vi "GUI_HTU_Chicane.vi"() -> ()   [LabVIEW 2013]
uses:
  Shared/GUI_Template/GUI_master/tcp_new_data_event.ctl
  Shared/GUI_Template/GUI_master/tcp new data cluster.ctl
panel:
  in  "DigitalOutput.Channel 5::4":enum16{"on", "off"}(ring) caption="ChicaneSlits\nplunger"
  in  "GUIdevice 4":string="U_Valve_Daq"
  in  "Ch1Ax2MovePos::3":bool=TRUE caption="Blank Button"
  in  "Ch1Ax2MoveNeg::3":bool=TRUE caption="Blank Button"
  in  "Ch1Ax1MovePos::3":bool=TRUE caption="Blank Button"
  in  "Ch1Ax1MoveNeg::3":bool=TRUE caption="Blank Button"
  in  "Ch1Ax2StepSize::3":dbl caption="High E Step size (mm)" min=0.01 max=2.0
  in  "Ch1Ax1StepSize::3":dbl caption="Low E Step size (mm)" min=0.01 max=2.0
  in  "Voltage::2":dbl caption="Inner \nVoltage" min=0.0 max=15.0
  in  "Current::2":dbl caption="Inner \nCurrent" min=-12.0 max=12.0
  in  "Voltage::1":dbl caption="Outer \nVoltage" min=0.0 max=15.0
  in  "Current::1":dbl caption="Outer \nCurrent" min=-12.0 max=12.0
  in  "Enable_Output::2":bool=TRUE caption="Blank Button"
  in  "Enable_Output::1":bool=TRUE caption="Blank Button"
  in  "GUIdevice 3":string="U_ChicaneMotors"
  in  "Enable_Output::2":enum16{"on", "off"}(ring) caption="Enable inner"
  in  "Enable_Output::1":enum16{"on", "off"}(ring) caption="Enable outer"
  in  "RunList::2":enum16{"on", "off"}(ring) caption="Run List \nInner Pair"
  in  "RunList::1":enum16{"on", "off"}(ring) caption="Run List \nOuter Pair"
  in  "LoadList::2":enum16{"on", "off"}(ring) caption="Load List \nInner Pair"
  in  "LoadList::1":enum16{"on", "off"}(ring) caption="Load List \nOuter Pair"
  out "Chart":cluster{"Value":dbl, "Value":dbl}(graph)
  in  "ApplyChicaneSettings":bool
  in  "Energy (MeV)":dbl=100.0
  in  "R56 (um)":dbl
  out "Offset (mm)":dbl
  out "Width of 2%  (mm)":dbl
  out "SetCurrent":dbl
  in  "CalculateChicaneSettings":bool
  out "error IO 2":errorcluster
  out "tcp data event":T1
  in  "UDP error message":string
  in  "GUIdevice 2":string="U_ChicaneInner"
  in  "GUIdevice 1":string="U_ChicaneOuter"
  in  "stop":bool
  # "HTU Chicane"
  # "Chicane slit operation"
  # "Energy"
  # "Outer pair"
  # "Inner pair"
  # "Enable"
  # "Current"
  # "Move High E direction"
  # "Voltage"
  # "Move Low E direction"
  # "Degaussing"
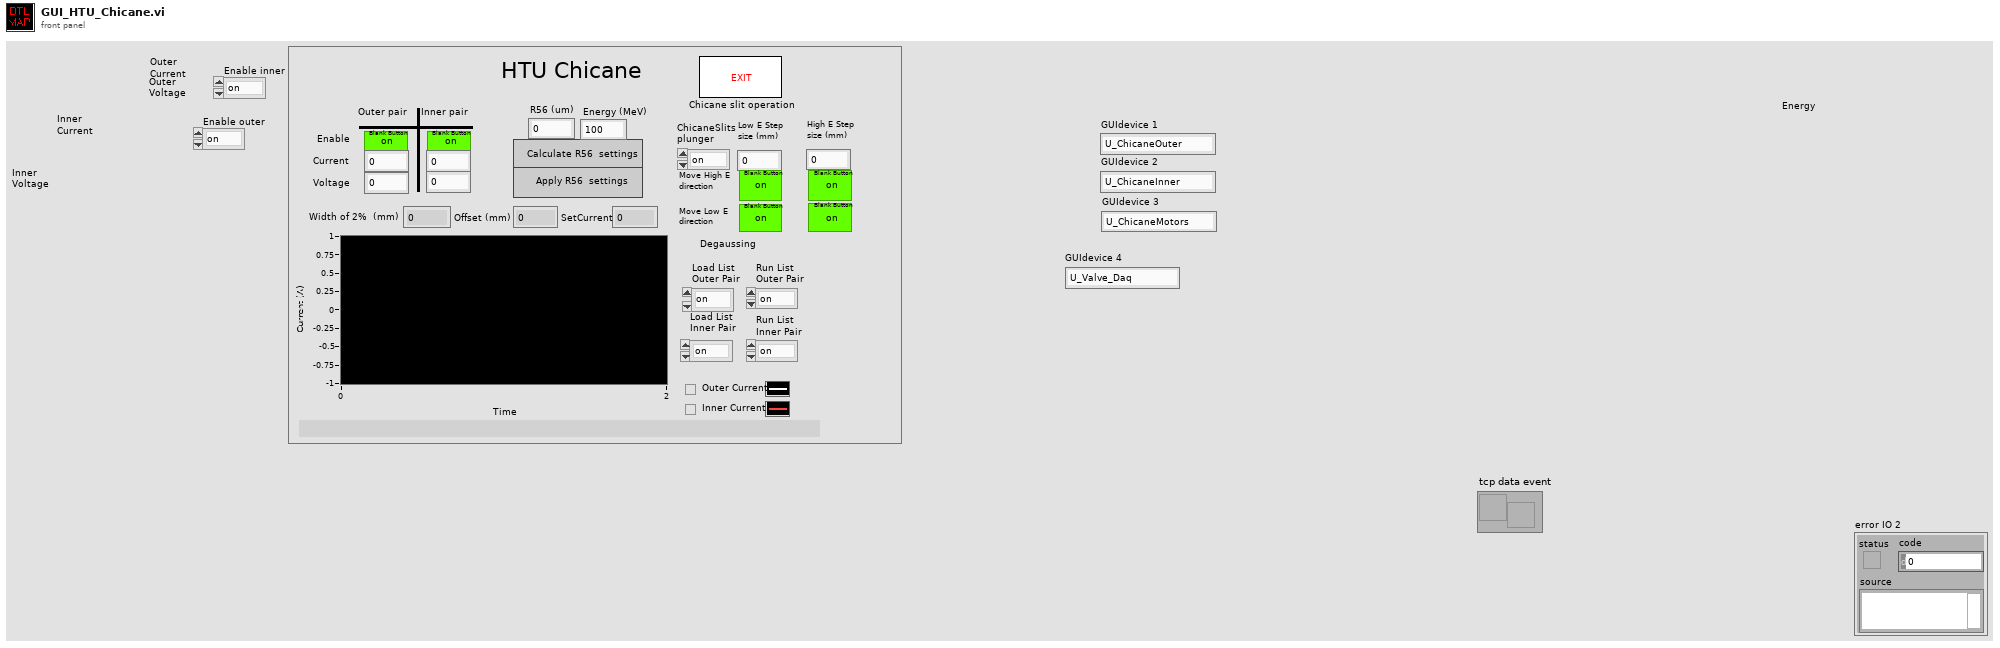
[diagram p1: front panel]
types:
  T1 = typedef "tcp_new_data_event.ctl" = refnum<user-event>
  T2 = typedef "tcp new data cluster.ctl" = cluster{"EventEnum":enum16{"new data", "connection status update"}, "Device name":string}
  T3 = enum32{"invalid app kind", "Development System", "Run Time System", "Student Edition", "Embedded LabVIEW", "Evaluation", "Custom"}
  T4 = enum32{"Invalid", "Standard", "Closed", "Hidden", "Minimized", "Maximized"}
  T5 = cluster{"Core":cluster{"Current VI Reference":refnum<vi>, "Close Panel on Exit?":bool}, "CalculateChicanceSettings":bool, "ApplyChicanceSettings":bool, "CurrentGraph1":dbl[][], "last chart update tck":i32}
  T6 = cluster{"Current VI Reference":refnum<vi>, "Close Panel on Exit?":bool}
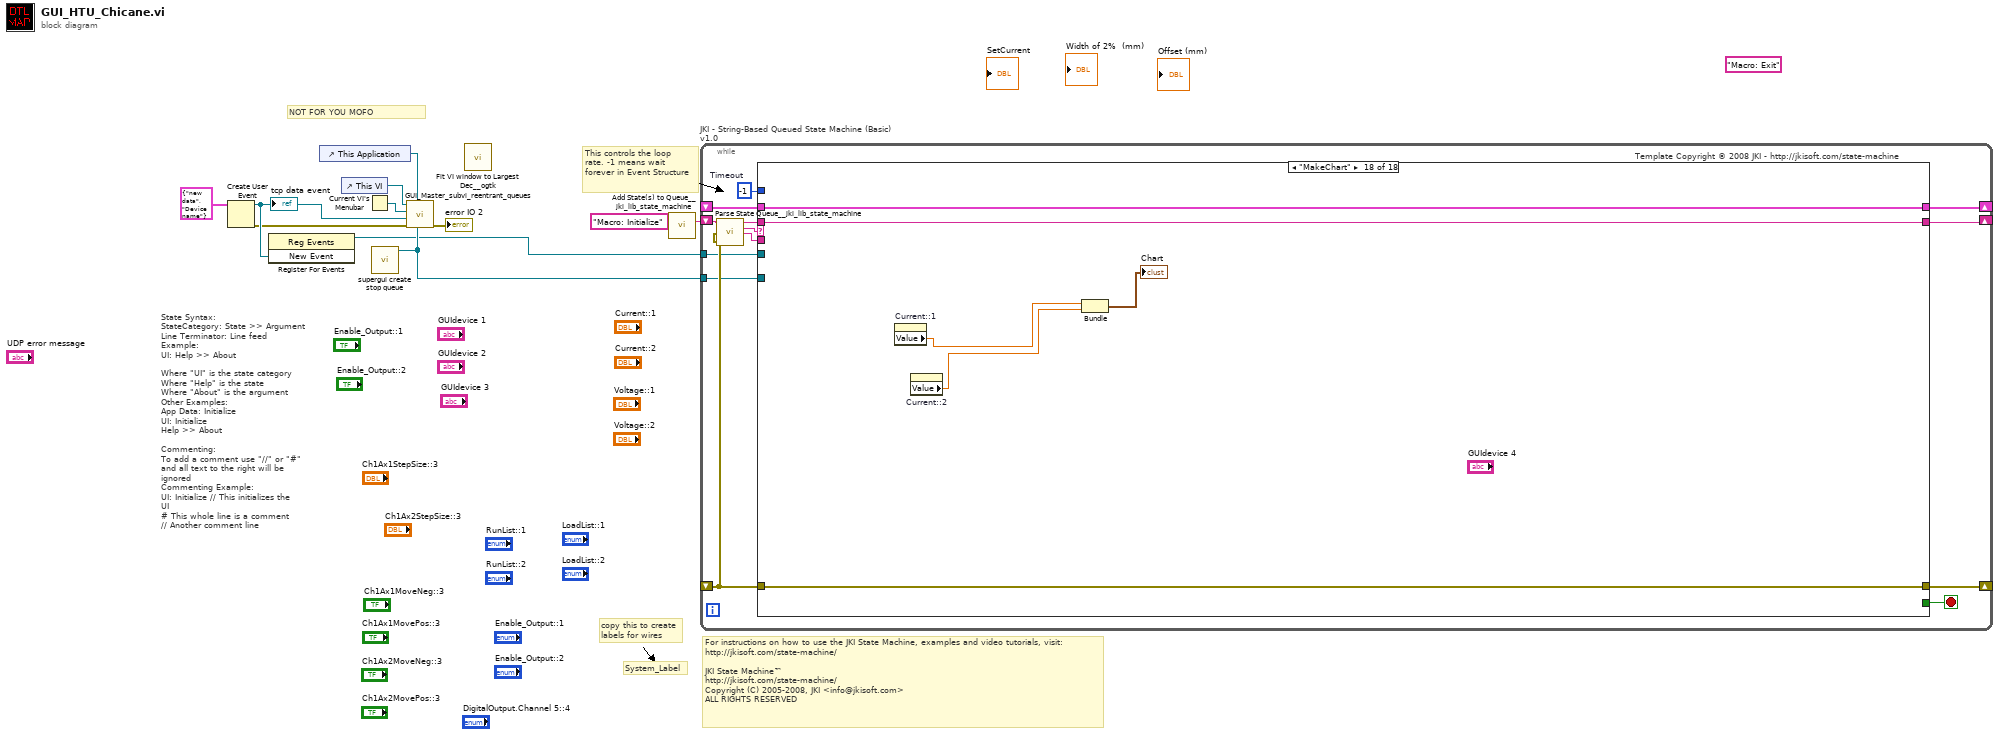
[diagram p0: block diagram]
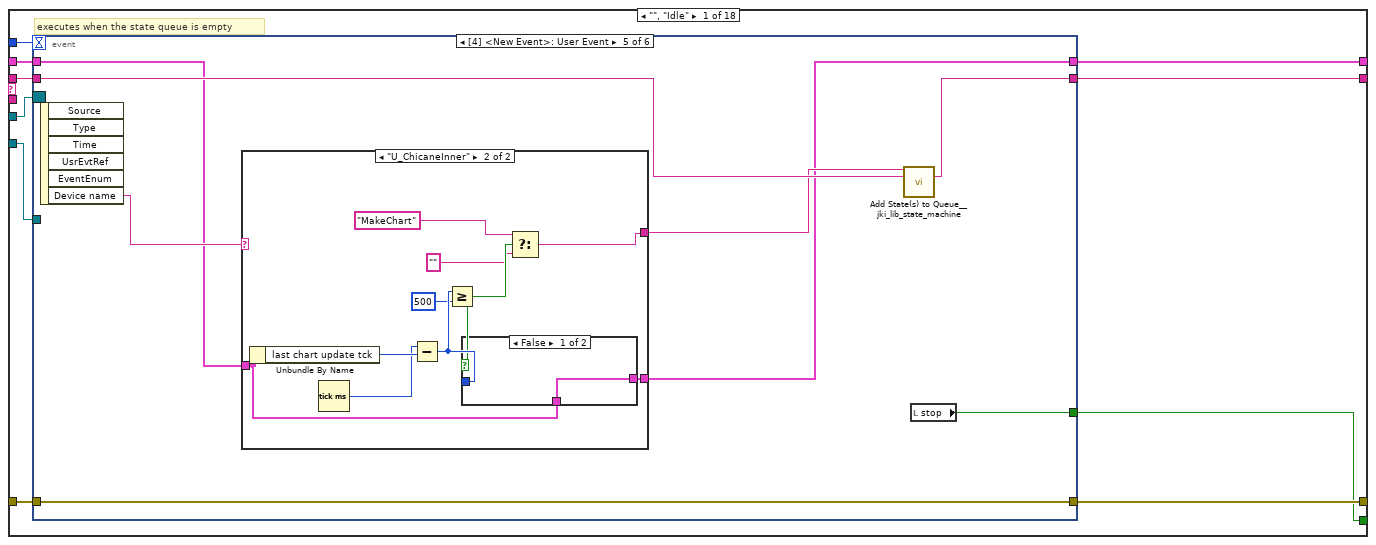
[diagram p2: hidden frame]
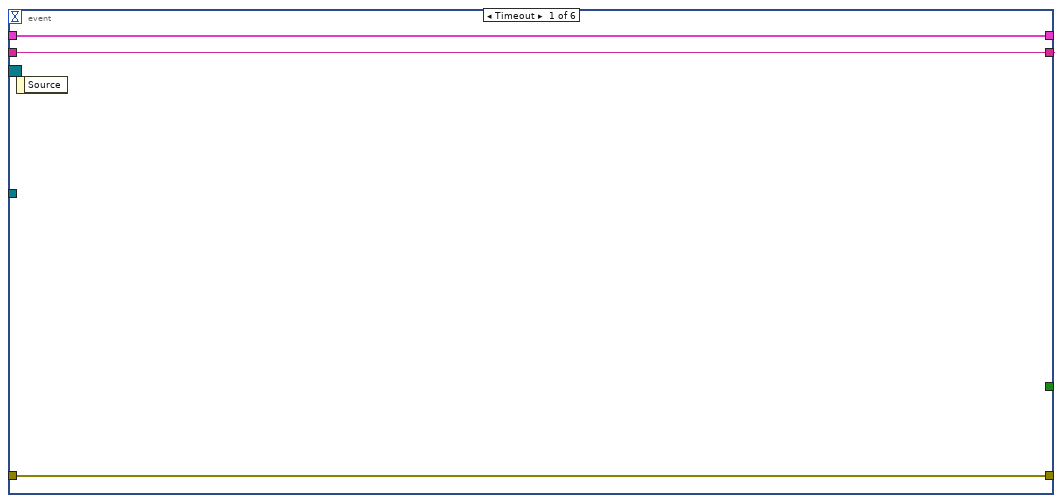
[diagram p3: hidden frame]
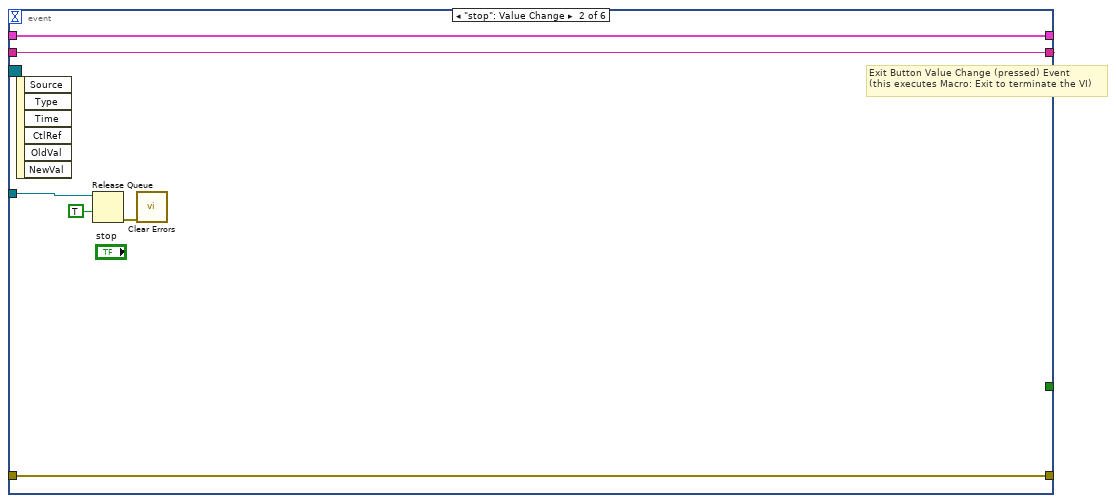
[diagram p4: hidden frame]
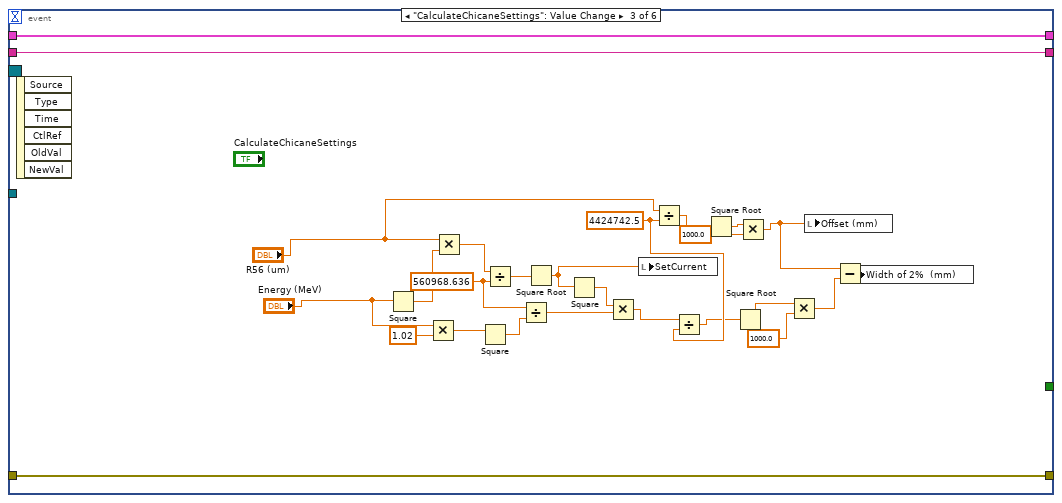
[diagram p5: hidden frame]
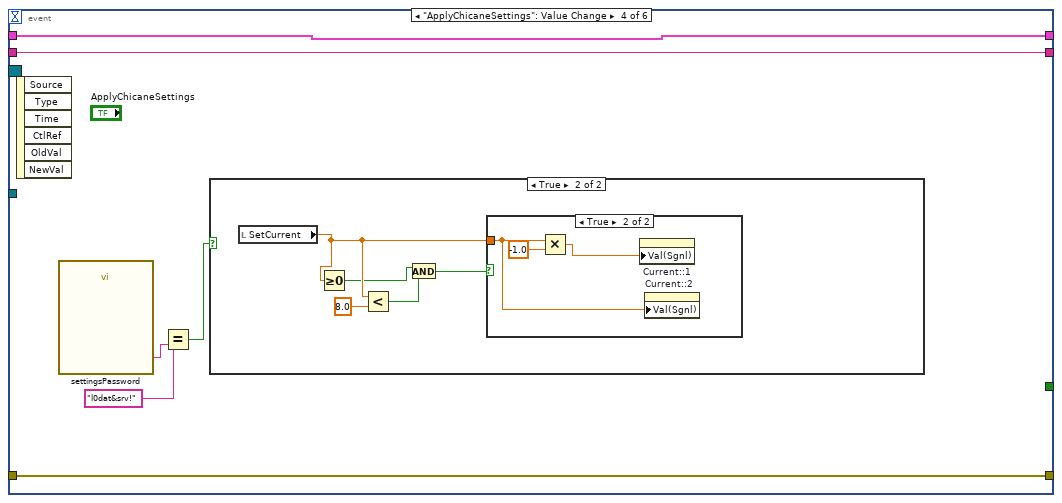
[diagram p6: hidden frame]
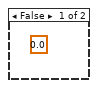
[diagram p7: hidden frame]
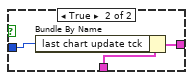
[diagram p10: hidden frame]
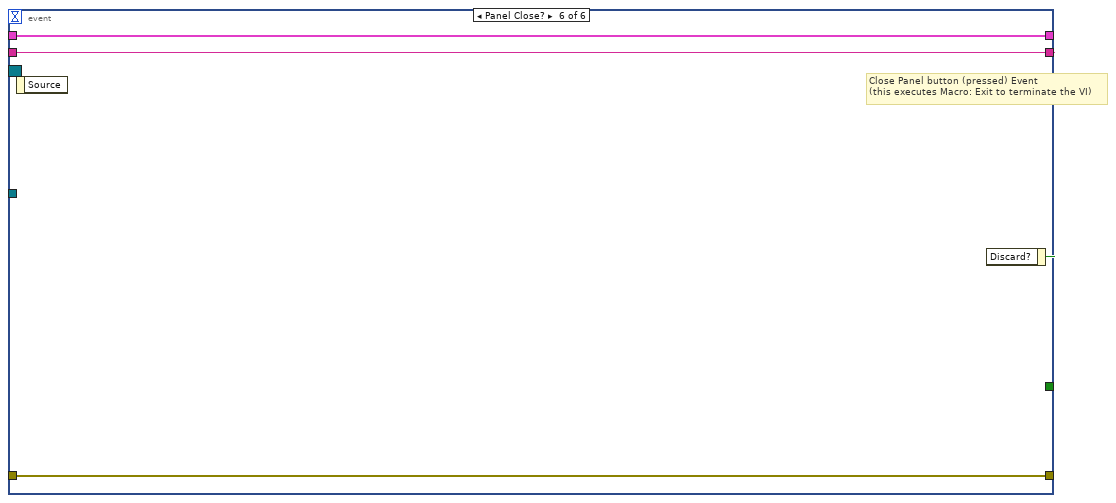
[diagram p11: hidden frame]
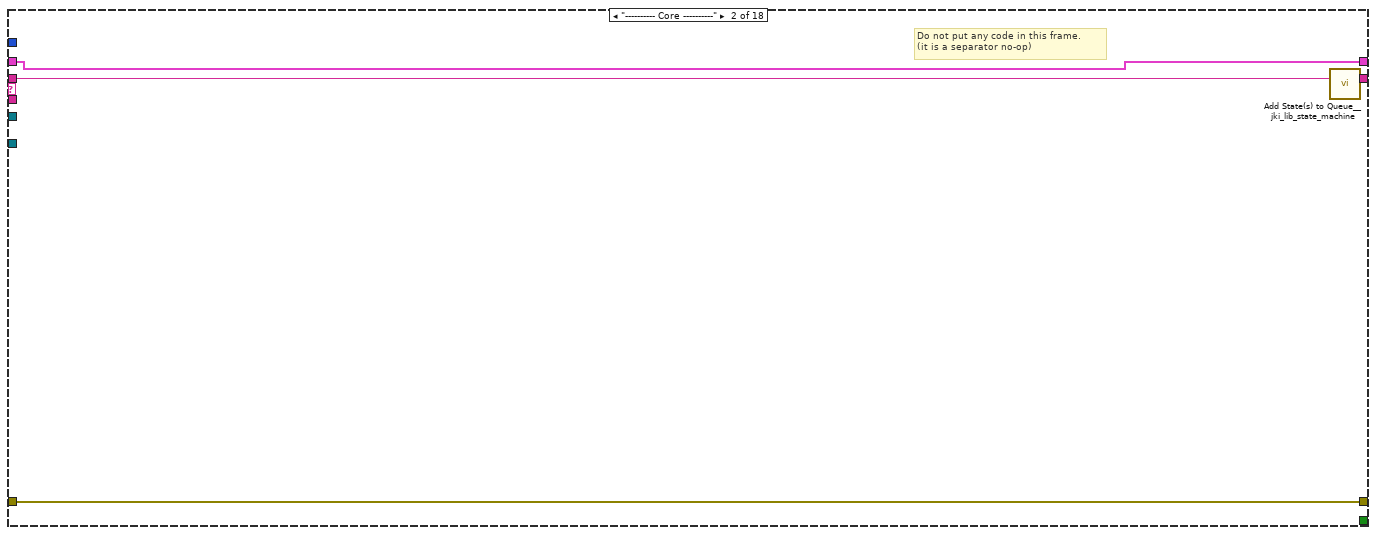
[diagram p12: hidden frame]
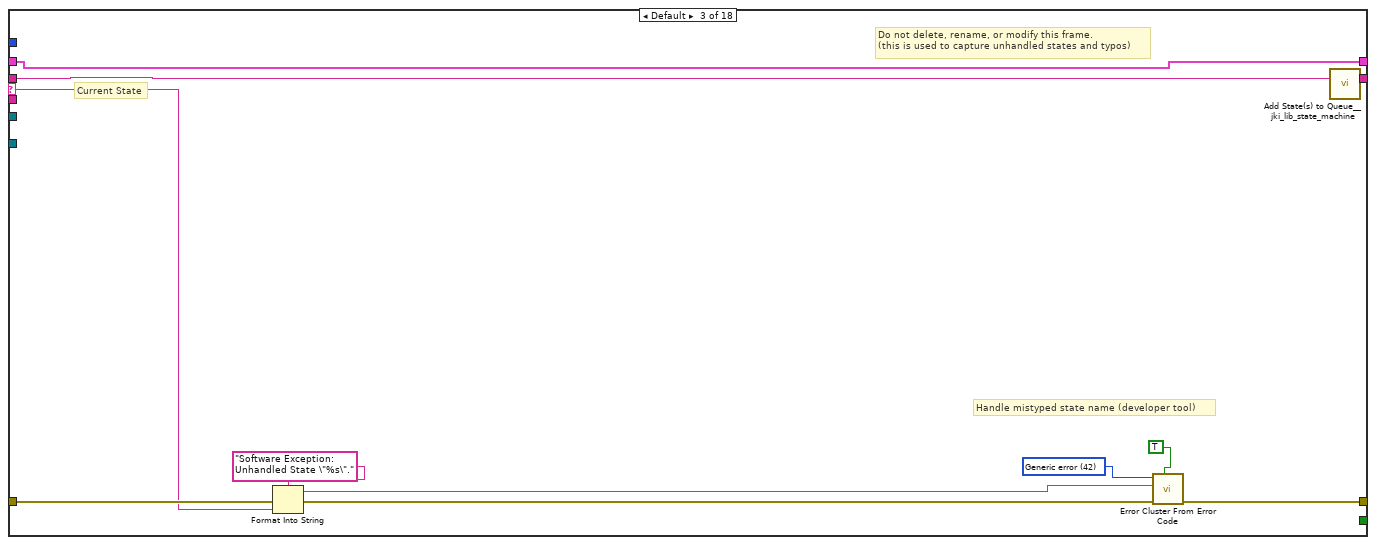
[diagram p13: hidden frame]
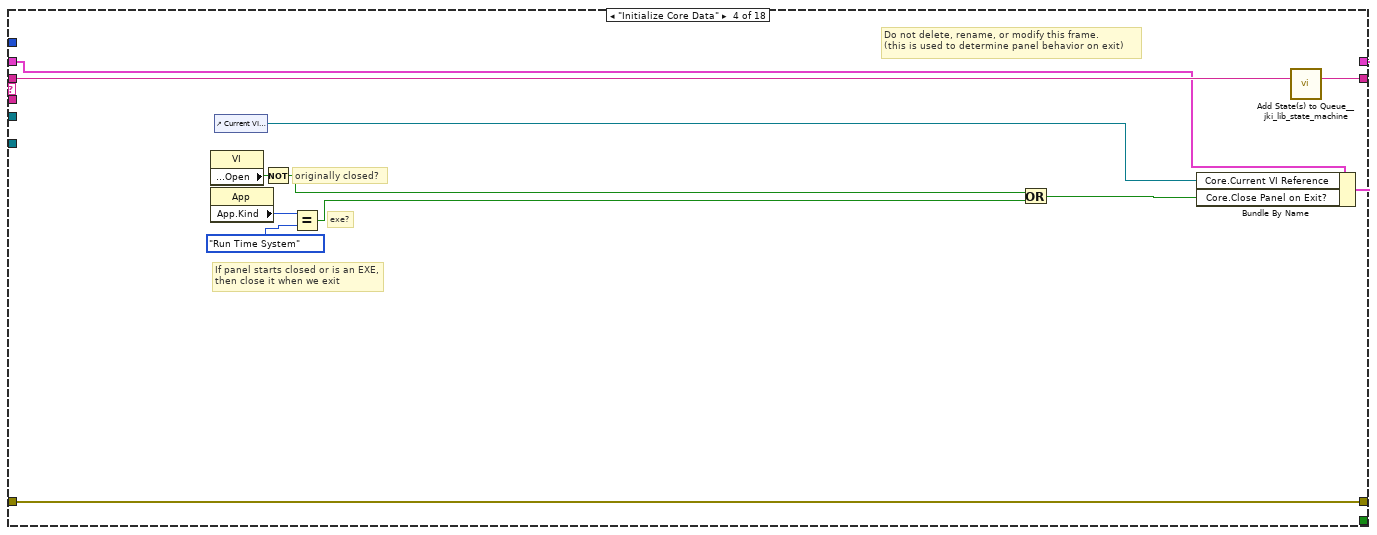
[diagram p14: hidden frame]
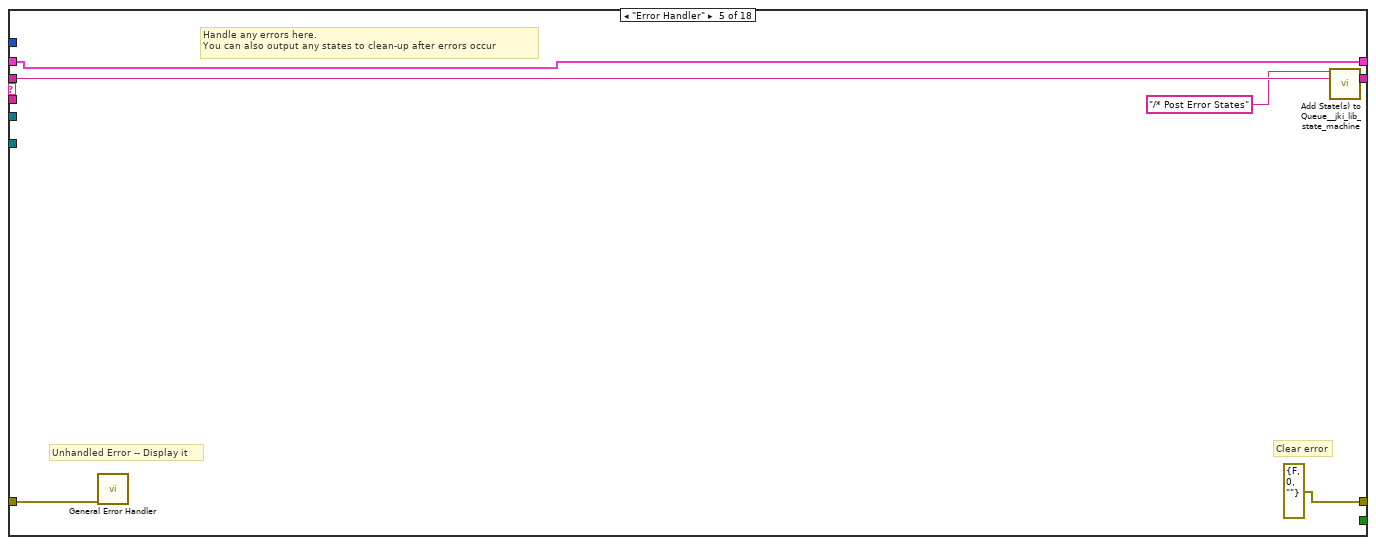
[diagram p15: hidden frame]
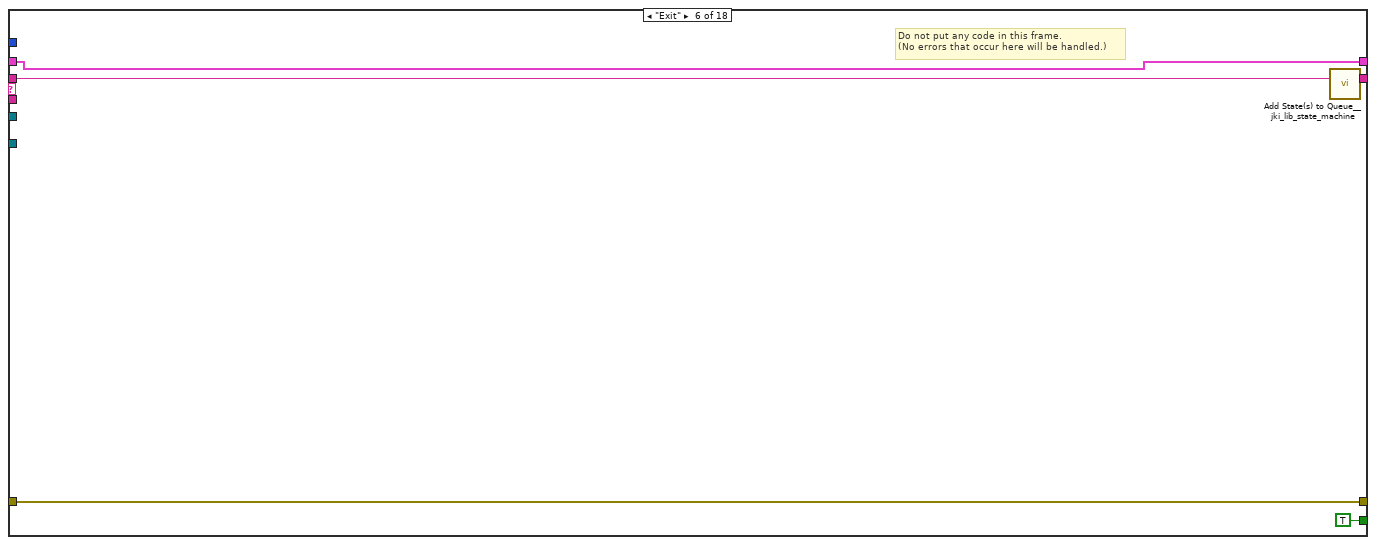
[diagram p16: hidden frame]
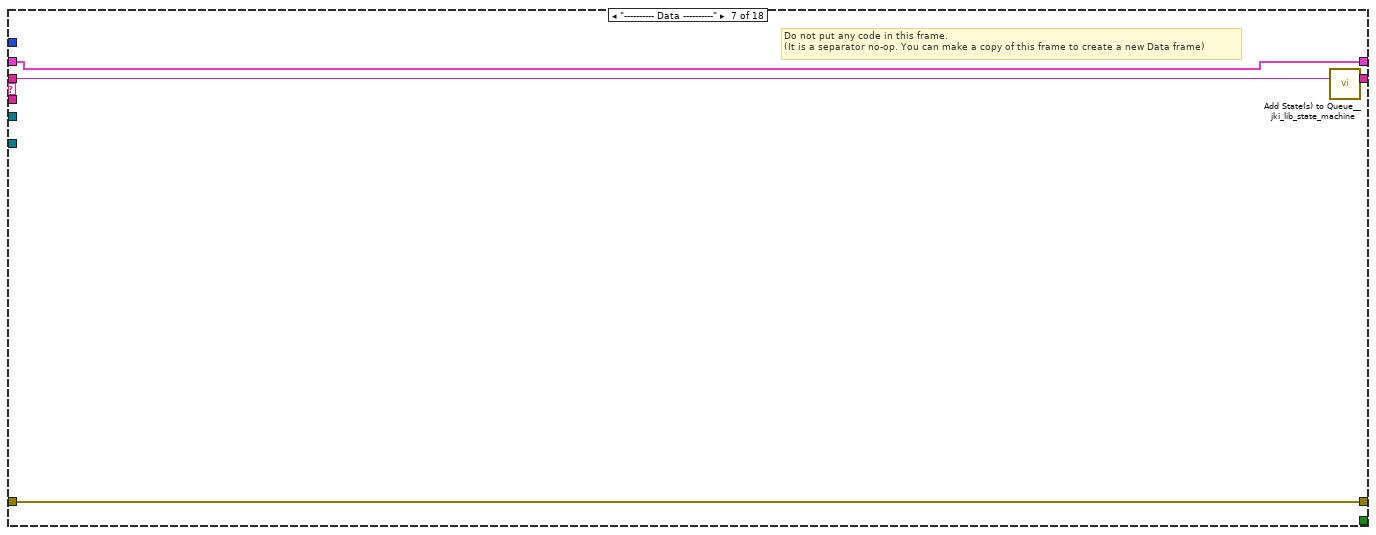
[diagram p17: hidden frame]
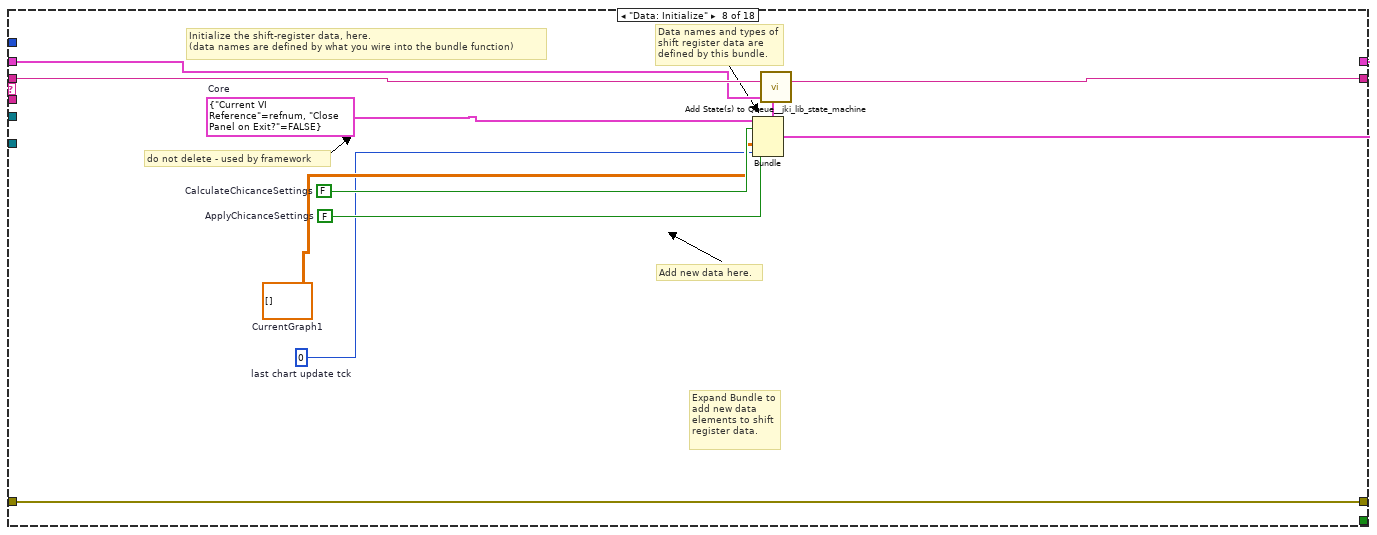
[diagram p18: hidden frame]
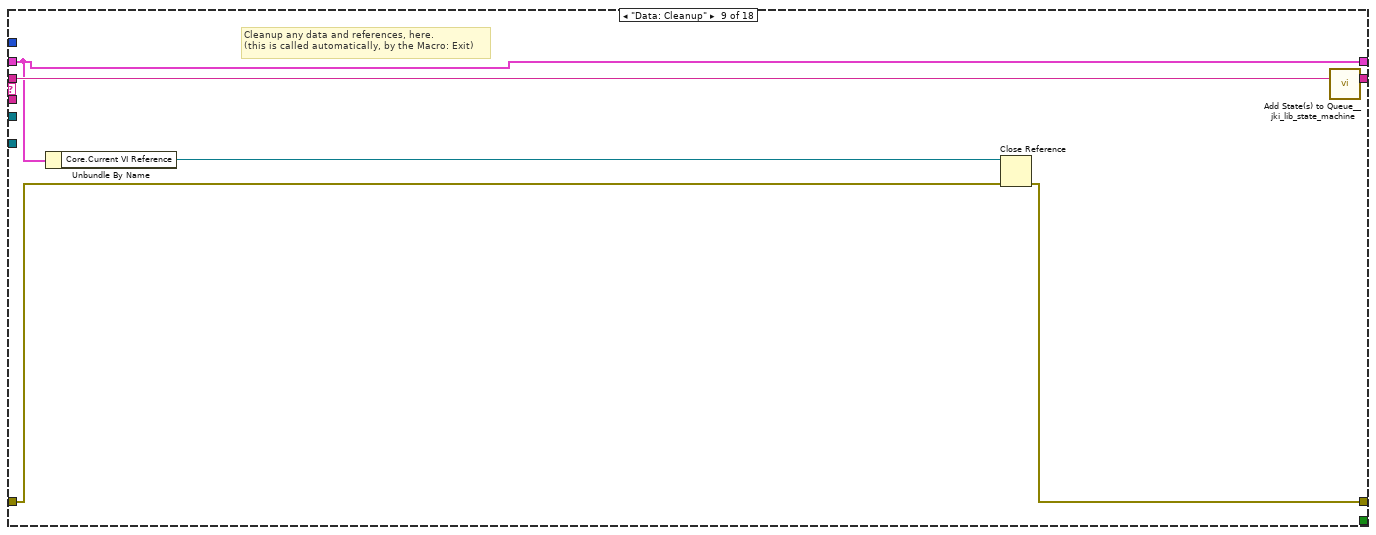
[diagram p19: hidden frame]
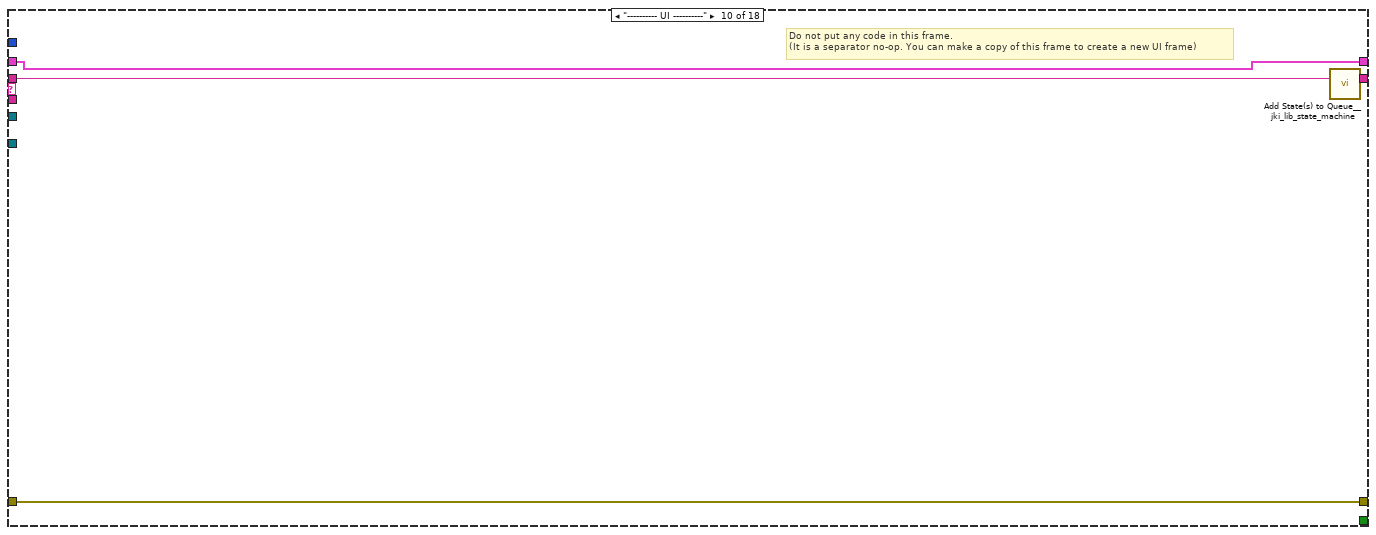
[diagram p20: hidden frame]
diagram:
  (unwired) "Macro: Exit"
  # "For instructions on how to use the JKI State Machine, examples and video tutorials, visit:\nhttp://jkisoft.com/state-machine/\n\nJKI State Machine™\nhttp://jkisoft.com/state-machine/\nCopyright (C) 2005-2008, JKI <info@jkisoft.com>\nALL RIGHTS RESERVED"
  # "State Syntax:\nStateCategory: State >> Argument\nLine Terminator: Line feed\nExample:\nUI: Help >> About\n\nWhere \"UI\" is the state category\nWhere \"Help\" is the state\nWhere \"About\" is the argument\nOther Examples:\nApp Data: Initialize\nUI: Initialize\nHelp >> About\n\nCommenting:\nTo add a comment use \"//\" or \"#\" and all text to the right will be ignored\nCommenting Example:\nUI: Initialize // This initializes the UI\n# This whole line is a comment\n// Another comment line"
  # "copy this to create labels for wires"
  # "This controls the loop rate. -1 means wait forever in Event Structure"
  # "System_Label"
  # "NOT FOR YOU MOFO"
  n1 = Create User Event(user event datatype=T2 {"EventEnum"=enum."new data", "Device name"="Device name"} ("New Event")) -> (user event=w10:refnum<user-event>, error out=w9:errorcluster)  [unwired: 1 in]
  "tcp data event" <- w10
  n2 = register-events(w10) -> (reference out=w1:refnum<event-registration>)  [unwired: 2 in, 1 out]
  n3 = control-ref of="This Application"() -> (w11:refnum<vi>)
  n4 = control-ref of="This VI"() -> (w5:refnum<vi>)
  n5 = Current VI's Menubar() -> (w7:refnum<k9>)
  n6 = call "supergui create stop queue.vi"() -> ("STOP Queue out"=w2:refnum<queue>)  [unwired: 11 in]
  n7 = call "GUI_Master_subvi_reentrant_queues.vi"("STOP Queue in"=w2, "This Application"=w11, "error in (no error)"=w9, "tcp data event"=w10, "Caller menu reference"=w7, "Caller VI ref"=w5) -> ("error out"=→"error IO 2":errorcluster)  [unwired: 5 in]
  n8 = call <userlib>:"Fit VI window to Largest Dec__ogtk.vi"() -> ()  [unwired: 6 in, 2 out]
  n9 = call <vilib>:"Add State(s) to Queue__jki_lib_state_machine.vi"("State(s) in (\"\")"="Macro: Initialize") -> ("States Out"=w3:string)  [unwired: 14 in]
  n10 = while "JKI - String-Based Queued State Machine (Basic) v1.0" {
    shift-right: [w17] -> _
    shift-left: _ -> [w16]
    shift-right: [w20] -> _
    shift-left: _ -> [w14]
    shift-right: [w19] -> _
    shift-left: w3 -> [w21]
    tunnel: w1 -> [w13]
    tunnel: w2 -> [w12]
    stop <- w18 stop-if-true
    w15 = -1  # Timeout
    # "Template Copyright © 2008 JKI - http://jkisoft.com/state-machine"
    n11 = call <vilib>:"Parse State Queue__jki_lib_state_machine.vi"("State Queue"=w21, "Error In (no error)"=w14) -> ("Remaining States"=w23:string, "Current State"=w24:string, "Arguments"=w22:string)  [unwired: 11 in]
    n12 = case shown="\"MakeChart\"" w24 {
      selector: w24 -> [_ _ w120 _ _ _ _ _ _ _ _ _ _ _ _ _ _ _]
      tunnel: w23 -> [w34 w119 w124 w142 w148 w153 w157 w167 w173 w177 w181 w187 w198 w224 w229 w239 w243 w248]
      tunnel: w22 -> [_ _ _ _ _ _ _ _ _ _ _ w182 w193 _ _ _ _ _]
      tunnel: w16 -> [w32 w116 w122 w132 w145 w151 w154 w162 w168 w174 w179 w185 w192 w221 w226 w230 w240 w249]
      tunnel: [w31 w117 w126 w140 errorcluster {"status"=FALSE, "code"=0, "source"=""} ("error out") w150 w155 w165 w170 w175 w178 w183 w195 w222 w227 w237 w241 w247] -> w20
      tunnel: w14 -> [w30 w117 w125 w140 w144 w150 w155 w165 w171 w175 w178 w184 w196 w222 w227 w237 w241 w247]
      tunnel: [w33 w118 w123 w141 w147 w152 w156 w166 w172 w176 w180 w186 w197 w223 w228 w238 w242 w248] -> w19
      tunnel: [w25 _ _ _ _ TRUE _ _ _ _ _ _ _ _ _ _ _ _] -> w18
      tunnel: [w26 w116 w122 w131 w145 w151 w154 w161 w168 w174 w179 w185 w192 w221 w226 w230 w240 w249] -> w17
      tunnel: w15 -> [w29 _ _ _ _ _ _ _ _ _ _ _ _ _ _ _ _ _]
      tunnel: w13 -> [w28 _ _ _ _ _ _ _ _ _ _ _ _ _ _ _ _ _]
      tunnel: w12 -> [w27 _ _ _ _ _ _ _ _ _ _ _ _ _ _ _ _ _]
      frame "", "Idle" {
        # "executes when the state queue is empty"
        n13 = event shown="[4] <New Event>: User Event" {
          selector: w28 -> [_ _ _ _ _ _]
          dyn-events: _ -> [_ _ _ _ _ _]
          timeout: w29 -> [_ _ _ _ _ _]
          tunnel: w34 -> [w38 w46 w72 w78 w93 w115]
          tunnel: [w37 w45 w72 w78 w91 w114] -> w33
          tunnel: w32 -> [w35 w43 w70 w74 w89 w112]
          tunnel: [w36 w44 w71 w77 w90 w113] -> w31
          tunnel: w30 -> [w36 w44 w71 w77 w90 w113]
          tunnel: [w35 w43 w70 w74 w88 w112] -> w26
          tunnel: w27 -> [_ w40 _ _ _ _]
          tunnel: [_ _ _ _ w87 _] -> w25
          event Timeout {
            n14 = event-data() -> ()  [unwired: 1 in, 1 out]
            n15 = call <vilib>:"Add State(s) to Queue__jki_lib_state_machine.vi"("State(s) in (\"\")"=w38) -> ("States Out"=w37:string)  [unwired: 14 in]
          }
          event "stop": Value Change {
            # "Exit Button Value Change (pressed) Event\n(this executes Macro: Exit to terminate the VI)"
            n16 = event-data() -> ()  [unwired: 1 in, 6 out]
            n17 = Release Queue(queue=w40, force destroy? (F)=TRUE) -> (error out=w41:errorcluster)  [unwired: 1 in, 2 out]
            n18 = call <vilib>:"Clear Errors.vi"("error in (no error)"=w41) -> ()  [unwired: 6 in, 1 out]
            n19 = call <vilib>:"Add State(s) to Queue__jki_lib_state_machine.vi"("State(s) in Front (\"\")"="Macro: Exit", "State(s) in (\"\")"=w46) -> ("States Out"=w45:string)  [unwired: 13 in]
          }
          event "CalculateChicaneSettings": Value Change {
            w53 = 4424742.5 ("y")
            w60 = 560968.636 ("y")
            n20 = event-data() -> ()  [unwired: 1 in, 6 out]
            n21 = Square(x="Energy (MeV)") -> (x^2=w55:dbl)
            n22 = Multiply(x="Energy (MeV)", y=1.02) -> (x*y=w59:dbl)
            n23 = Multiply(x="R56 (um)", y=w55) -> (x*y=w56:dbl)
            n24 = Square(x=w59) -> (x^2=w61:dbl)
            n25 = Divide(x=w56, y=w60) -> (x/y=w65:dbl)
            n26 = Divide(x=w60, y=w61) -> (x/y=w62:dbl)
            n27 = Square Root(x=w65) -> (sqrt(x)=w66:dbl)
            n28 = Square(x=w66) -> (x^2=w63:dbl)
            n29 = Multiply(x=w63, y=w62) -> (x*y=w54:dbl)
            n30 = local write "SetCurrent"(w66) -> ()
            n31 = Divide(x="R56 (um)", y=w53) -> (x/y=w67:dbl)
            n32 = Divide(x=w54, y=w53) -> (x/y=w52:dbl)
            n33 = Square Root(x=w67) -> (sqrt(x)=w69:dbl)
            n34 = Square Root(x=w52) -> (sqrt(x)=w51:dbl)
            n35 = Multiply(x=w69, y=1000.0) -> (x*y=w49:dbl)
            n36 = Multiply(x=w51, y=1000.0) -> (x*y=w48:dbl)
            n37 = local write "Offset (mm)"(w49) -> ()
            n38 = Subtract(x=w49, y=w48) -> (x-y=w47:dbl)
            n39 = local write "Width of 2%  (mm)"(w47) -> ()
          }
          event "ApplyChicaneSettings": Value Change {
            n40 = event-data() -> ()  [unwired: 1 in, 6 out]
            n41 = call "settingsPassword.vi"() -> ("password"=w76:string)  [unwired: 17 in, 2 out]
            n42 = Equal?(x="l0dat&srv!", y=w76) -> (x = y?=w73:bool)
            n43 = case shown="True" w73 {
              frame False {
                (unwired) 0.0 ("opening Time")
              }
              frame True {
                n44 = local read "SetCurrent"() -> (w83:dbl)
                n45 = Greater Or Equal To 0?(x=w83) -> (x >= 0?=w81:bool)
                n46 = Less?(x=w83, y=8.0) -> (x < y?=w80:bool)
                n47 = And(x=w81, y=w80) -> (x .and. y?=w79:bool)
                n48 = case shown="True" w79 {
                  tunnel: w83 -> [_ w84]
                  frame False {
                  }
                  frame True {
                    n49 = Multiply(x=w84, y=-1.0) -> (x*y=w85:dbl)
                    n50 = property on="Current::1" class="DigNum (strict)"("Val(Sgnl)"=w85) -> ()  [unwired: 2 in, 2 out]
                    n51 = property on="Current::2" class="DigNum (strict)"("Val(Sgnl)"=w84) -> ()  [unwired: 2 in, 2 out]
                  }
                }
              }
            }
          }
          event User Event {
            n52 = event-data() -> ("Device name"=w94:string)  [unwired: 1 in, 5 out]
            n53 = case shown="\"U_ChicaneInner\"" w94 {
              tunnel: [_ w96] -> w92
              tunnel: w89 -> [w95 w101]
              tunnel: [w95 w100] -> w88
              frame "False", Default {
              }
              frame "U_ChicaneInner" {
                n54 = Unbundle By Name(w101) -> ("last chart update tck"=w105:i32)
                n55 = Tick Count (ms)() -> (millisecond timer value=w104:u32)
                n56 = Subtract(x=w104, y=w105) -> (x-y=w103:u32)
                n57 = Greater Or Equal?(x=w103, y=u32 500) -> (x >= y?=w98:bool)
                n58 = case shown="False" w98 {
                  tunnel: w103 -> [_ w108]
                  tunnel: w101 -> [w106 w109]
                  tunnel: [w106 w107] -> w100
                  frame False {
                  }
                  frame True {
                    n59 = Bundle By Name(cluster=w109, "last chart update tck"=w108) -> (w107:T5)
                  }
                }
                n60 = Select(t="MakeChart", s=w98, f="") -> (s? t:f=w96:string)
              }
            }
            n61 = call <vilib>:"Add State(s) to Queue__jki_lib_state_machine.vi"("State(s) in Front (\"\")"=w92, "State(s) in (\"\")"=w93) -> ("States Out"=w91:string)  [unwired: 13 in]
            n62 = local read "stop"() -> (w87:bool)
          }
          event Panel Close? {
            # "Discard the event because we'll close the front panel ourselves in Macro: Exit"
            # "Close Panel button (pressed) Event\n(this executes Macro: Exit to terminate the VI)"
            n63 = event-data() -> ()  [unwired: 1 in, 1 out]
            n64 = event-data("Discard?"=TRUE) -> ()  [unwired: 1 in, 1 out]
            n65 = call <vilib>:"Add State(s) to Queue__jki_lib_state_machine.vi"("State(s) in Front (\"\")"="Macro: Exit", "State(s) in (\"\")"=w115) -> ("States Out"=w114:string)  [unwired: 13 in]
          }
        }
      }
      frame "---------- Core ----------" {
        # "Do not put any code in this frame.\n(it is a separator no-op)"
        n66 = call <vilib>:"Add State(s) to Queue__jki_lib_state_machine.vi"("State(s) in (\"\")"=w119) -> ("States Out"=w118:string)  [unwired: 14 in]
      }
      frame Default {
        w129 = 42 items=["No error", "Argument error", "Memory is full", "Out of zone", "End of file", "File already open", "Generic file I/O error", "File not found", "File permission error", "Disk is full", "Duplicate path", "Too many files open", "System feature not enabled", "Resource file not found", "Cannot add resource", "Resource not found", "Image not found", "Image memory error", "Pen does not exist", "Config type invalid", "Config token not found", "Config parse error", "Config memory error", "Bad external code format", "Bad external code offset", "External code not present", "Null window", "Destroy window error", "Null menu", "Print aborted", "Bad print record", "Print driver error", "Windows error during printing", "Memory error during printing", "Print dialog error", "Generic print error", "Invalid device refnum", "Device not found", "Device parameter error", "Device unit error", "Cannot open device", "Device call aborted", "Generic error", "Cancelled by user", "Object ID too low", "Object ID too high", "Object not in heap", "Unknown heap", "Unknown object (invalid DefProc)", "Unknown object (DefProc not in table)", "Message out of range", "Invalid (null) method", "Unknown message", "Manager call not supported", "Bad address", "Network operation in progress", "Network operation timed out", "Connection is busy", "Network attribute not supported", "Network error", "Address in use", "System out of memory", "Connection aborted", "Connection refused", "Not connected", "Already connected", "Connection closed", "Initialization error (interapplication manager)", "Bad occurrence", "Wait on unbound occurrence handler", "Occurrence queue overflow", "Datalog type conflict", "Unused", "Unrecognized type (interapplication manager)", "Memory corrupt", "Failed to make temporary DLL", "Old CIN version", "Drag socket not found", "Failed to load drop-object", "Failed to register OLE object", "Failed to release OLE object", "Format specifier type mismatch", "Unknown format specifier", "Too few format specifiers", "Too many format specifiers", "Scan failed", "Newer CIN version", "Error converting to variant", "Runtime menu error", "Password tampered", "Variant attribute not found", "Incompatible variant data type", "Event data is not available", "Event Store is not present", "Occurrence is not found", "Event Queue is not created", "Event info is not available", "Refnum passed is NULL", "Error retrieving Class GUID", "Error retrieving CoClass GUID", "Error retrieving TypeLib GUID.", "Bad built application magic bytes.", "Specific driver is different from the specific driver associated with the Logical Name.", "There is no session opened to the class driver.", "Max Error", "MAX - Error with config objects", "MAX - Error loading configuration", "MAX - Group not supported"]
        # "Current State"
        # "Do not delete, rename, or modify this frame.\n(this is used to capture unhandled states and typos)"
        # "Handle mistyped state name (developer tool)"
        n67 = Format Into String(format string="Software Exception: Unhandled State \"%s\"." ("message"), error in=w125, w120) -> (resulting string=w128:string, error out=w127:errorcluster)  [unwired: 1 in]
        n68 = call <vilib>:"Error Cluster From Error Code.vi"("show call chain? (False)"=TRUE, "error in (no error)"=w127, "error message (\"\")"=w128, "error code (0)"=w129) -> ("error out"=w126:errorcluster)  [unwired: 5 in]
        n69 = call <vilib>:"Add State(s) to Queue__jki_lib_state_machine.vi"("State(s) in (\"\")"=w124) -> ("States Out"=w123:string)  [unwired: 14 in]
      }
      frame "Initialize Core Data" {
        # "Do not delete, rename, or modify this frame.\n(this is used to determine panel behavior on exit)"
        # "originally closed?"
        # "exe?"
        # "If panel starts closed or is an EXE, then close it when we exit"
        n70 = property class="VI"() -> ("Front Panel.Open"=w139:bool)  [unwired: 2 in, 2 out]
        n71 = property class="App"() -> ("App.Kind"=w138:T3)  [unwired: 2 in, 2 out]
        n72 = control-ref of="Current VI Reference"() -> (w133:refnum<vi>)
        n73 = Not(x=w139) -> (.not. x?=w136:bool)
        n74 = Equal?(x=w138, y=T3."Run Time System" ("Application:Kind")) -> (x = y?=w135:bool)
        n75 = Or(x=w136, y=w135) -> (x .or. y?=w134:bool)
        n76 = Bundle By Name(cluster=w132, "Core.Current VI Reference"=w133, "Core.Close Panel on Exit?"=w134) -> (w131:T5)
        n77 = call <vilib>:"Add State(s) to Queue__jki_lib_state_machine.vi"("State(s) in (\"\")"=w142) -> ("States Out"=w141:string)  [unwired: 14 in]
      }
      frame "Error Handler" {
        # "Unhandled Error -- Display it"
        # "Handle any errors here.\nYou can also output any states to clean-up after errors occur"
        # "Clear error"
        n78 = call <vilib>:"General Error Handler.vi"("error in (no error)"=w144) -> ()  [unwired: 10 in, 5 out]
        n79 = call <vilib>:"Add State(s) to Queue__jki_lib_state_machine.vi"("State(s) in Front (\"\")"="/* Post Error States", "State(s) in (\"\")"=w148) -> ("States Out"=w147:string)  [unwired: 13 in]
      }
      frame "Exit" {
        # "Do not put any code in this frame.\n(No errors that occur here will be handled.)"
        n80 = call <vilib>:"Add State(s) to Queue__jki_lib_state_machine.vi"("State(s) in (\"\")"=w153) -> ("States Out"=w152:string)  [unwired: 14 in]
      }
      frame "---------- Data ----------" {
        # "Do not put any code in this frame.\n(It is a separator no-op. You can make a copy of this frame to create a new Data frame)"
        n81 = call <vilib>:"Add State(s) to Queue__jki_lib_state_machine.vi"("State(s) in (\"\")"=w157) -> ("States Out"=w156:string)  [unwired: 14 in]
      }
      frame "Data: Initialize" {
        w158 = 0  # last chart update tck
        w159 = dbl[][] []  # CurrentGraph1
        w160 = FALSE  # ApplyChicanceSettings
        w163 = FALSE  # CalculateChicanceSettings
        w164 = T6 {"Current VI Reference"=refnum, "Close Panel on Exit?"=FALSE}  # Core
        # "do not delete - used by framework"
        # "Expand Bundle to add new data elements to shift register data."
        # "Add new data here."
        # "Data names and types of shift register data are defined by this bundle."
        # "Initialize the shift-register data, here.\n(data names are defined by what you wire into the bundle function)"
        n82 = Bundle(cluster=w162, "Core"=w164, "CalculateChicanceSettings"=w163, "ApplyChicanceSettings"=w160, "CurrentGraph1"=w159, "last chart update tck"=w158) -> (w161:T5)
        n83 = call <vilib>:"Add State(s) to Queue__jki_lib_state_machine.vi"("State(s) in (\"\")"=w167) -> ("States Out"=w166:string)  [unwired: 14 in]
      }
      frame "Data: Cleanup" {
        # "Cleanup any data and references, here.\n(this is called automatically, by the Macro: Exit)"
        n84 = Unbundle By Name(w168) -> ("Core.Current VI Reference"=w169:refnum<vi>)
        n85 = Close Reference(reference=w169, error in (no error)=w171) -> (error out=w170:errorcluster)
        n86 = call <vilib>:"Add State(s) to Queue__jki_lib_state_machine.vi"("State(s) in (\"\")"=w173) -> ("States Out"=w172:string)  [unwired: 14 in]
      }
      frame "---------- UI ----------" {
        # "Do not put any code in this frame.\n(It is a separator no-op. You can make a copy of this frame to create a new UI frame)"
        n87 = call <vilib>:"Add State(s) to Queue__jki_lib_state_machine.vi"("State(s) in (\"\")"=w177) -> ("States Out"=w176:string)  [unwired: 14 in]
      }
      frame "UI: Initialize" {
        # "Initialize the User Interface, here.\n(this is called automatically, by the Macro: Init)"
        n88 = call <vilib>:"Add State(s) to Queue__jki_lib_state_machine.vi"("State(s) in (\"\")"=w181) -> ("States Out"=w180:string)  [unwired: 14 in]
      }
      frame "UI: Cursor Set" {
        # "Argument"
        # "Set and Unset Cursor Busy.\n(Usage: \"UI: Cursor Set >> Busy|Idle\")"
        n89 = case shown="\"Idle\", Default" w182 {
          tunnel: w184 -> [w189 w191]
          tunnel: [w188 w190] -> w183
          frame "Idle", Default {
            n90 = call <vilib>:"Unset Busy.vi"("error in (no error)"=w189) -> ("error out"=w188:errorcluster)  [unwired: 10 in]
          }
          frame "Busy" {
            n91 = call <vilib>:"Set Busy.vi"("error in (no error)"=w191) -> ("error out"=w190:errorcluster)  [unwired: 9 in, 1 out]
          }
        }
        n92 = call <vilib>:"Add State(s) to Queue__jki_lib_state_machine.vi"("State(s) in (\"\")"=w187) -> ("States Out"=w186:string)  [unwired: 14 in]
      }
      frame "UI: Front Panel State" {
        # "Argument"
        # "Set Front Panel Open or Closed\n(Usage: \"UI: Front Panel State >> Open|Close\")"
        n93 = Unbundle By Name(w192) -> ("Core.Current VI Reference"=w194:refnum<vi>)
        n94 = case shown="\"Open\", Default" w193 {
          tunnel: w196 -> [w203 w215]
          tunnel: [w204 w216] -> w195
          tunnel: w194 -> [w199 w211]
          frame "Open", Default {
            n95 = property class="VI"(reference=w199, error in=w203) -> (reference out=w201:refnum<vi>, error out=w202:errorcluster, "Front Panel.Open"=w200:bool)
            n96 = case shown="False" w200 {
              tunnel: [w207 w210] -> w204
              tunnel: w202 -> [w206 w210]
              tunnel: w201 -> [w205 _]
              frame False {
                n97 = invoke class="VI" method="FP.Open"(reference=w205, error in=w206, "Activate"=TRUE, "State"=T4."Standard") -> (error out=w207:errorcluster)  [unwired: 1 in, 4 out]
              }
              frame True {
              }
            }
          }
          frame "Close" {
            n98 = property class="VI"(reference=w211, error in=w215) -> (reference out=w213:refnum<vi>, error out=w214:errorcluster, "Front Panel.Open"=w212:bool)
            n99 = case shown="True" w212 {
              tunnel: [w217 w220] -> w216
              tunnel: w214 -> [w217 w219]
              tunnel: w213 -> [_ w218]
              frame False {
              }
              frame True {
                n100 = invoke class="VI" method="FP.Close"(reference=w218, error in=w219) -> (error out=w220:errorcluster)  [unwired: 1 in, 2 out]
              }
            }
          }
        }
        n101 = call <vilib>:"Add State(s) to Queue__jki_lib_state_machine.vi"("State(s) in (\"\")"=w198) -> ("States Out"=w197:string)  [unwired: 14 in]
      }
      frame "---------- Macro ----------" {
        # "Do not put any code in this frame.\n(It is a separator no-op. You can make a copy of this frame to create a new Macro frame)"
        n102 = call <vilib>:"Add State(s) to Queue__jki_lib_state_machine.vi"("State(s) in (\"\")"=w224) -> ("States Out"=w223:string)  [unwired: 14 in]
      }
      frame "Macro: Initialize" {
        w225 = "Data: Initialize\nInitialize Core Data\nUI: Initialize\nUI: Front Panel State >> Open"  # Data: Initialize Initialize Core Data UI: Initialize UI: Front Panel State >> Open
        # "Initialization Macro\n(This is called once, when the VI starts)"
        n103 = call <vilib>:"Add State(s) to Queue__jki_lib_state_machine.vi"("State(s) in Front (\"\")"=w225, "State(s) in (\"\")"=w229) -> ("States Out"=w228:string)  [unwired: 13 in]
      }
      frame "Macro: Exit" {
        # "Exit Macro\n(This is called once, when the VI exits)"
        n104 = Unbundle By Name(w230) -> ("Core.Close Panel on Exit?"=w231:bool)
        n105 = Select(t="UI: Front Panel State >> Close", s=w231, f="") -> (s? t:f=w234:string)
        n106 = call <vilib>:"Add State(s) to Queue__jki_lib_state_machine.vi"("State(s) in (\"\")"=w234, "State(s) at Back (\"\")"="Data: Cleanup\nExit") -> ("States Out"=w232:string)  [unwired: 13 in]
        n107 = call <vilib>:"Add State(s) to Queue__jki_lib_state_machine.vi"("State(s) in Front (\"\")"=w232, "State(s) in (\"\")"=w239) -> ("States Out"=w238:string)  [unwired: 13 in]
      }
      frame "---------- New Category ----------" {
        # "Template Separator\n(You can make a copy of, or modify, this frame)"
        n108 = call <vilib>:"Add State(s) to Queue__jki_lib_state_machine.vi"("State(s) in (\"\")"=w243) -> ("States Out"=w242:string)  [unwired: 14 in]
      }
      frame "MakeChart" {
        n109 = property on="Current::1" class="DigNum (strict)"() -> ("Value"=w246:dbl)  [unwired: 2 in, 2 out]
        n110 = property on="Current::2" class="DigNum (strict)"() -> ("Value"=w245:dbl)  [unwired: 2 in, 2 out]
        n111 = Bundle("Value"=w246, "Value"=w245) -> (→"Chart":cluster{"Value":dbl, "Value":dbl})  [unwired: 1 in]
      }
    }
  }
